vi "FTW-ScheduledJob-Initialize.vi"(0 "FTW Scheduled Job":refnum<class "FTW-ScheduledJob.lvclass">, 5 "Identity":string, 7 "Job":string, 9 "Iterations (-1 to loop forever)":i32=-1 format="%d iterations", 11 "error in":errorcluster) -> (4 "FTW Scheduled Job out":refnum<class "FTW-ScheduledJob.lvclass">, 15 "error out":errorcluster)   [LabVIEW 2015, in "FTW-ScheduledJob.lvclass"]
uses:
  FTW-ScheduledJob.lvclass
panel:
  # "Inputs"
  # "Outputs"
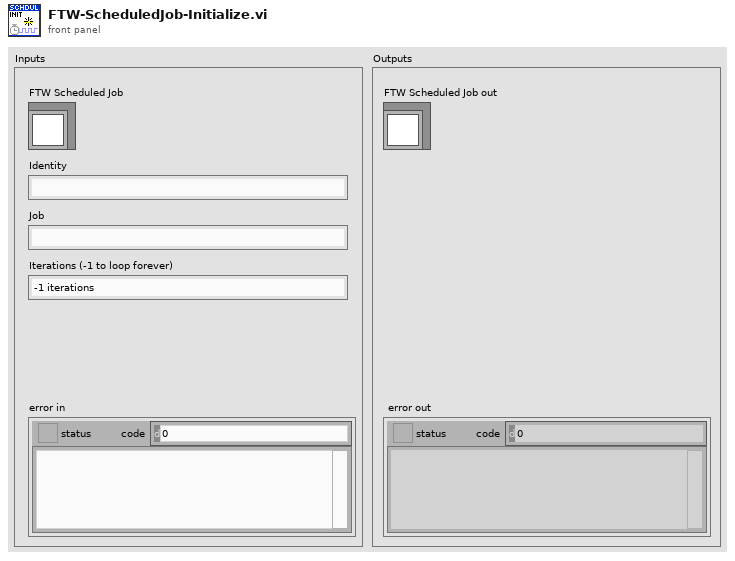
[diagram p1: front panel]
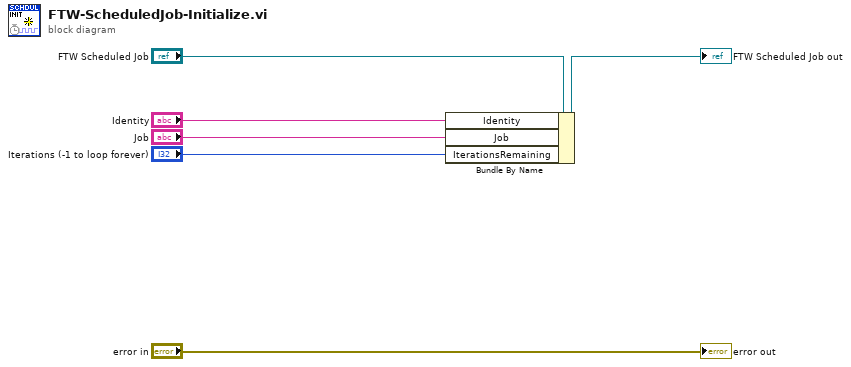
[diagram p0: block diagram]
diagram:
  n1 = Bundle By Name(cluster="FTW Scheduled Job", "Identity"="Identity", "Job"="Job", "IterationsRemaining"="Iterations (-1 to loop forever)") -> (→"FTW Scheduled Job out":refnum<class "FTW-ScheduledJob.lvclass">)
  "error out" <- "error in"
